vi "Write Setpoint_ref.vi"(8 "error in (no error)":errorcluster, 10 "setpoint ref":refnum<vi>, 11 "Y_H in":refnum<class "Y_H.lvclass">) -> (0 "error out":errorcluster, 3 "Y_H out":refnum<class "Y_H.lvclass">)   [LabVIEW 2019, in "Y_H.lvclass"]
uses:
  Y_H.lvclass
  Y_H.lvclass/Y_H.ctl
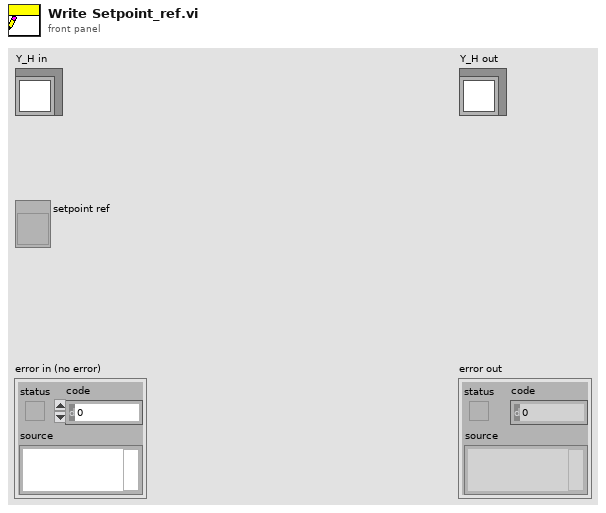
[diagram p1: front panel]
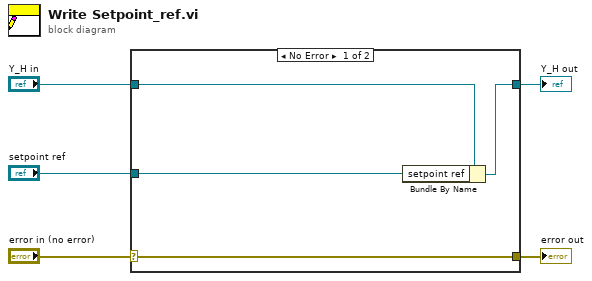
[diagram p0: block diagram]
diagram:
  n1 = case shown="No Error" "error in (no error)" {
    selector: "error in (no error)" -> [w9 w10]
    tunnel: [w9 w10] -> w4
    tunnel: [w7 w11] -> w2
    tunnel: "Y_H in" -> [w8 w11]
    tunnel: "setpoint ref" -> [w6 _]
    frame No Error {
      n2 = Bundle By Name(cluster=w8, "setpoint ref"=w6) -> (w7:refnum<class "Y_H.lvclass">)
    }
    frame Error {
    }
  }
  "error out" <- w4
  "Y_H out" <- w2
